vi "声卡.vi"() -> ()   [LabVIEW 2019]
uses:
  <vilib>/sound2/lvsound2.llb/Sound Input Read (DBL).vi
  <vilib>/express/express analysis/Spectral/Block/exnSpectralBlock spectral measurements RMS poly.vi
  <vilib>/express/express analysis/Spectral/Block/exnSpectralBlock spectral measurements RMS WFM.vi
  <vilib>/express/express analysis/Spectral/XNode/ExpressSpectralMeasurementsBlockNode.xnode
  <vilib>/Analysis/NI_AALPro.lvlib
panel:
  in  "停止按钮":bool
  out "频谱（Express节点）":cluster{"f0":dbl, "df":dbl, "magnitude":dbl[]}(graph)
  out "频谱（APS函数）":T1(graph)
  out "原始时域":waveform(dbl)[](graph)
  in  "采样模式":u32(ring) items=["", "连续采样", "单次采样"]
  in  "声音格式":cluster{"采样率":dbl, "通道数":dbl, "每采样比特数":dbl}
  in  "设备id":u32(ring) items=["1", "0"]
  in  "每通道采样数":i32
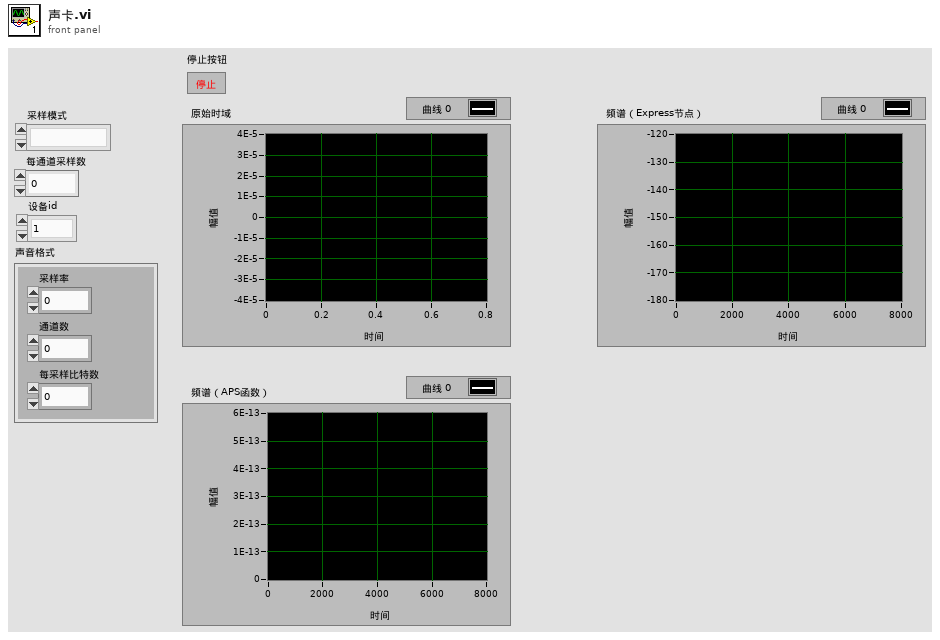
[diagram p1: front panel]
types:
  T1 = cluster{i32, "df":dbl, "Power Spectrum (V^2 rms)":dbl[]}
  T2 = typedef "Sound Input Task ID.ctl" = u32
  T3 = cluster{"averaging mode":u16, "weighting mode":u16, "number of averages":u32}
  T4 = cluster{"dB On (F)":bool, "unwrap phase (F)":bool, "convert to degree (F)":bool}
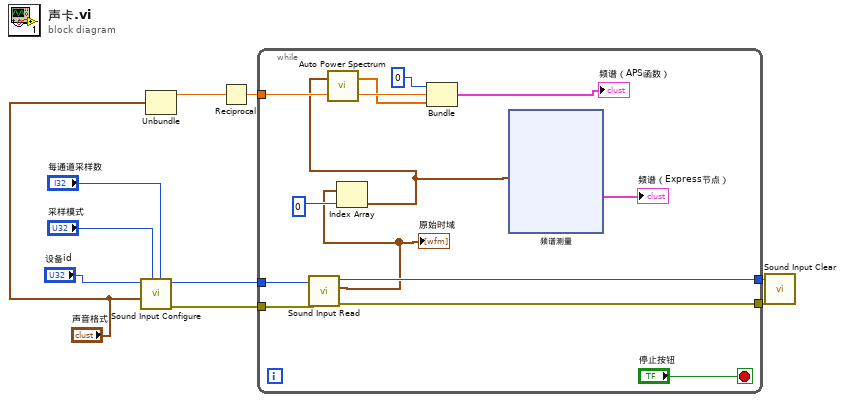
[diagram p0: block diagram]
diagram:
  n1 = call <vilib>:"Sound Input Configure.vi"("number of samples/ch"="每通道采样数", "sample mode"="采样模式", "sound format"="声音格式", "device ID"="设备id") -> ("error out"=w3:errorcluster, "task ID"=w4:T2)  [unwired: 6 in]
  n2 = Unbundle("声音格式") -> ("采样率"=w6:dbl)  [unwired: 2 out]
  n3 = Reciprocal(x=w6) -> (1/x=w5:dbl)
  n4 = while {
    tunnel: w5 -> [w24]
    tunnel: w4 -> [w23]
    tunnel: w3 -> [w22]
    tunnel: [w21] -> w2
    tunnel: [w20] -> w1
    stop <- "停止按钮" stop-if-true
    n5 = call-poly <vilib>:"Sound Input Read.vi"("error in (no error)"=w22, "task ID"=w23) -> ("error out"=w20:errorcluster, "data"=w18:waveform(dbl)[], "task ID out"=w21:T2)  [unwired: 7 in]
    "原始时域" <- w18
    n6 = Index Array(array=w18, index=0) -> (element=w17:waveform(dbl))
    n7 = call <vilib>:"Auto Power Spectrum.vi"("dt"=w24, "Signal (V)"=w17) -> ("df"=w15:dbl, "Power Spectrum (V^2 rms)"=w14:dbl[])
    n8 = Bundle(0, "df"=w15, "Power Spectrum (V^2 rms)"=w14) -> (→"频谱（APS函数）":T1)  [unwired: 1 in]
    n9 = xnode "频谱测量"("信号"=w17) -> ("FFT - （均方根）"=→"频谱（Express节点）":cluster{"f0":dbl, "df":dbl, "magnitude":dbl[]})  [unwired: 1 in, 2 out]
  }
  n10 = call <vilib>:"Sound Input Clear.vi"("error in (no error)"=w1, "task ID"=w2) -> ()  [unwired: 9 in, 1 out]
